vi "test Factory.vi"() -> ()   [LabVIEW 2009]
uses:
  Analyze Classes/Analyze.lvlib
panel:
  out "Array 2":string[](array[string])
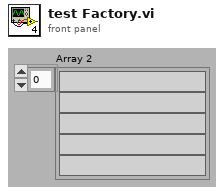
[diagram p1: front panel]
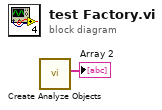
[diagram p0: block diagram]
diagram:
  n1 = call "Create Analyze Objects.vi"() -> ("Array 2"=→"Array 2":string[])  [unwired: 11 in]
